vi "Get proto Style Names.vi"(11 "Input Name":string) -> (3 "Proto Names":T1={"PascalCase"="Plugin8", "snake_case"="plugin_8"})   [LabVIEW 2021, in "Plugin Generator.lvlib"]
uses:
  Plugin Generator.lvlib
  Typedef/Proto Names.ctl
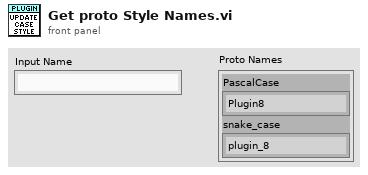
[diagram p1: front panel]
types:
  T1 = typedef "Plugin Generator.lvlib/Proto Names.ctl" = cluster{"PascalCase":string, "snake_case":string}
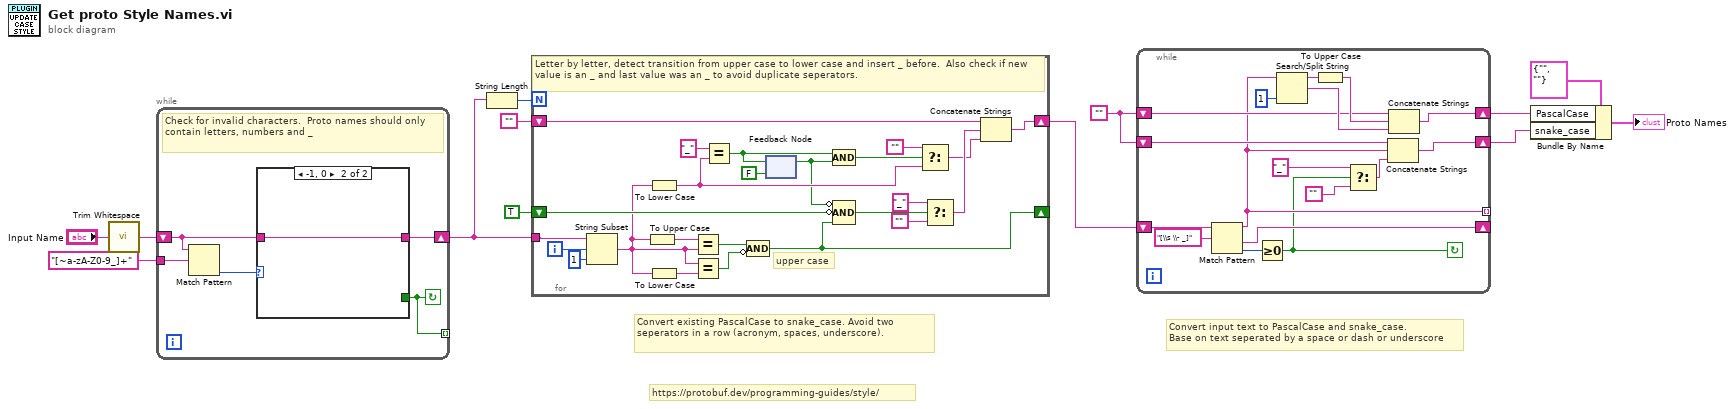
[diagram p0: block diagram]
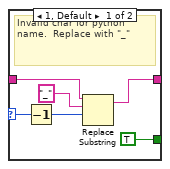
[diagram p2: hidden frame]
diagram:
  w13 = ""
  # "https://protobuf.dev/programming-guides/style/"
  # "Convert existing PascalCase to snake_case. Avoid two seperators in a row (acronym, spaces, underscore)."
  # "Convert input text to PascalCase and snake_case.\nBase on text seperated by a space or dash or underscore"
  n1 = call <vilib>:"Trim Whitespace.vi"("string"="Input Name") -> ("trimmed string"=w2:string)  [unwired: 1 in]
  n2 = while {
    tunnel: "[~a-zA-Z0-9_]+" ("regular expression") -> [w18]
    shift-right: [w15] -> w1
    shift-left: w2 -> [w16]
    tunnel: [w14] -> _ mode=indexing
    stop <- w14 continue-if-true
    # "Check for invalid characters.  Proto names should only contain letters, numbers and _"
    n3 = Match Pattern(string=w16, regular expression=w18) -> (offset past match=w17:i32)  [unwired: 1 in, 3 out]
    n4 = case shown="-1, 0" w17 {
      selector: w17 -> [w22 _]
      tunnel: w16 -> [w21 w25]
      tunnel: [w20 w25] -> w15
      tunnel: [TRUE _] -> w14
      frame 1, Default {
        # "Invalid char for python name.  Replace with \"_\""
        n5 = Decrement(x=w22) -> (x-1=w24:i32)
        n6 = Replace Substring(3:w24, 4:"_" ("substring (\"\")"), 5:w21) -> (1:w20:string)  [unwired: 1 in, 1 out]
      }
      frame -1, 0 {
      }
    }
  }
  n7 = String Length(string=w1) -> (length=w10:i32)
  n8 = for {
    N: w10 -> [_]
    tunnel: w1 -> [w49]
    shift-right: [w40] -> w8
    shift-left: "" -> [w46]
    shift-right: [w36] -> _
    shift-left: TRUE -> [w39]
    i -> [w48]
    # "upper case"
    # "Letter by letter, detect transition from upper case to lower case and insert _ before.  Also check if new value is an _ and last value was an _ to avoid duplicate seperators."
    n9 = String Subset(string=w49, offset (0)=w48, length (rest)=1 ("length (rest)")) -> (substring=w38:string)
    n10 = To Upper Case(1:w38) -> (0:w45:string)
    n11 = To Lower Case(string=w38) -> (all lower case string=w31:string)
    n12 = To Lower Case(string=w38) -> (all lower case string=w43:string)
    n13 = Equal?(x=w45, y=w38) -> (x = y?=w42:bool)
    n14 = Equal?(x=w38, y=w43) -> (x = y?=w41:bool)
    n15 = Equal?(x="_" ("regular expression"), y=w31) -> (x = y?=w29:bool)
    n16 = Compound Arithmetic op=AND(w42, invert w41) -> (w36:bool)
    n17 = feedback-in #1(w29) -> ()
    n18 = feedback #1(FALSE) -> (w28:bool)
    n19 = Compound Arithmetic op=AND(w29, w28) -> (w33:bool)
    n20 = Compound Arithmetic op=AND(invert w28, invert w39, w36) -> (w35:bool)
    n21 = Select(t="", s=w33, f=w31) -> (s? t:f=w32:string)
    n22 = Select(t="_", s=w35, f="") -> (s? t:f=w37:string)
    n23 = Concatenate Strings(w46, w37, w32) -> (w40:string)
  }
  n24 = while {
    tunnel: [w55] -> _ mode=indexing
    shift-right: [w63] -> _
    shift-left: w8 -> [w66]
    shift-right: [w51] -> w5
    shift-left: w13 -> [w56]
    shift-right: [w57] -> w6
    shift-left: w13 -> [w58]
    stop <- w53 continue-if-true
    n25 = Match Pattern(string=w66, regular expression="[\\s \\- _]") -> (before substring=w55:string, after substring=w63:string, offset past match=w64:i32)  [unwired: 1 in, 1 out]
    n26 = Greater Or Equal To 0?(x=w64) -> (x >= 0?=w53:bool)
    n27 = Search/Split String(string=w55, offset (0)=1) -> (substring before match=w61:string, match + rest of string=w59:string)  [unwired: 1 in, 1 out]
    n28 = To Upper Case(1:w61) -> (0:w60:string)
    n29 = Select(t="_", s=w53, f="") -> (s? t:f=w54:string)
    n30 = Concatenate Strings(w56, w55, w54) -> (w51:string)
    n31 = Concatenate Strings(w58, w60, w59) -> (w57:string)
  }
  n32 = Bundle By Name(cluster=T1 {"PascalCase"="", "snake_case"=""} ("Proto Names 2"), "PascalCase"=w6, "snake_case"=w5) -> (→"Proto Names":T1)
